vi "Instrument Do Core.vi"(8 "error in (no error)":errorcluster, 9 "Instrument in":refnum<class "Instrument Driver.lvclass">, 10 "Actor in":refnum<class "Actor.lvclass">, 11 "DMM Config Trigger Msg in":refnum<class "DMM Config Trigger Msg.lvclass">) -> (0 "error out":errorcluster, 1 "Instrument out":refnum<class "Instrument Driver.lvclass">, 2 "Actor out":refnum<class "Actor.lvclass">, 3 "DMM Config Trigger Msg out":refnum<class "DMM Config Trigger Msg.lvclass">, 5 "Data":refnum<class "Data.lvclass">)   [LabVIEW 2020, in "DMM Msg.lvlib" / "DMM Config Trigger Msg.lvclass"]
doc: "Set the trigger configuration on the DMM and return the Success boolean in a generic Boolean class."
uses:
  DMM Config Trigger Msg.lvclass
  PPL/HDH.Actor Framework.Core.Actor.lvlibp/1abvi3w/vi.lib/ActorFramework/Actor/Actor.lvclass
  PPL/HDH.Data.Generic.lvlibp/Data.lvclass
  PPL/HDH.Actor Framework.Core.Instrument Driver.lvlibp/Instrument Driver/Instrument Driver.lvclass
  PPL/HDH.Driver.DMM.lvlibp/DMM Driver.lvclass
  C:/Current projects/WS/PPL/HDH.Actor Framework.Core.Instrument Driver.lvlibp/Instrument Driver/Instrument Driver.lvclass
  DMM Config Trigger Msg.lvclass/DMM Config Trigger Msg.ctl
  PPL/HDH.Data.Generic.lvlibp/Generic Data/Boolean/Boolean.lvclass
  C:/Current projects/WS/PPL/HDH.Data.Generic.lvlibp/Data.lvclass
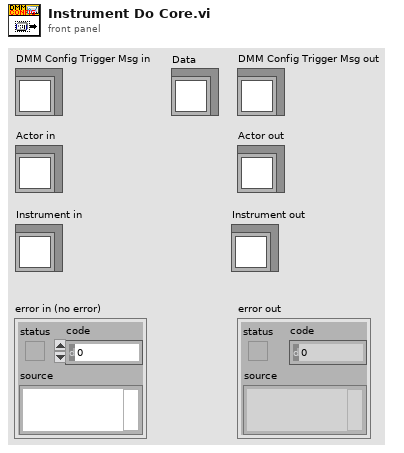
[diagram p1: front panel]
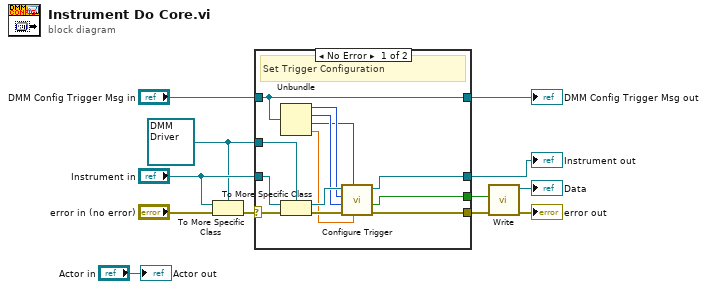
[diagram p0: block diagram]
diagram:
  w5 = refnum<class "DMM Driver.lvclass"> refnum ("HDH.Driver.DMM.lvlibp:DMM Driver.lvclass")
  n1 = To More Specific Class(target class=w5, reference="Instrument in", error in="error in (no error)") -> (error out=w10:errorcluster)  [unwired: 1 out]
  n2 = case shown="No Error" w10 {
    selector: w10 -> [w24 w27]
    tunnel: [w19 w27] -> w1
    tunnel: [w17 w26] -> w9
    tunnel: "DMM Config Trigger Msg in" -> [w17 w26]
    tunnel: [w18 w25] -> w7
    tunnel: "Instrument in" -> [w23 w25]
    tunnel: w5 -> [w22 _]
    tunnel: [w16 _] -> w3
    frame No Error {
      # "Set Trigger Configuration"
      n3 = Unbundle(w17) -> (w15:i32, w14:i32, w13:u16, w12:dbl)
      n4 = To More Specific Class(target class=w22, reference=w23, error in=w24) -> (specific class reference=w21:refnum<class "DMM Driver.lvclass">, error out=w20:errorcluster)
      n5 = call-dynamic "Configure Trigger.vi"("Sample Interval (-1s)"=w12, "Trigger Type Index(0)"=w13, "error in (no error)"=w20, "Samples per Trigger(1)"=w14, "Triggers to measure(1)"=w15, "DMM Driver in"=w21) -> ("error out"=w19:errorcluster, "Success?"=w16:bool, "DMM Driver out"=w18:refnum<class "DMM Driver.lvclass">)  [unwired: 3 in]
    }
    frame Error {
      # "Incorrect instrument - Return error"
    }
  }
  "error out" <- w1
  "DMM Config Trigger Msg out" <- w9
  "Instrument out" <- w7
  n6 = call "Write.vi"("Boolean"=w3) -> ("Boolean out"=→"Data":refnum<class "Boolean.lvclass">)  [unwired: 10 in]
  "Actor out" <- "Actor in"
